vi "DPT Panel Volume Size.vi"(0 "Default Volume Value":dbl, 11 "Error In":errorcluster) -> (4 "Scale Temp Coeff Out":dbl, 6 "Drum Volume":dbl=6.0, 8 "Out Strings":string[][](array[string]), 10 "MA Filter Size":i32=5, 15 "Error Out":errorcluster)   [LabVIEW 2016]
uses:
  Utility/Custom Pallet Controls/Custom Pallet Forward.ctl
  Utility/Custom Pallet Controls/Custom Pallet DBL.ctl
panel:
  in  "Drum Thermal\nVolume (>0)":T1=13.0 format="%.2f"
  in  "Tab Control":enum32{"Page 1", "Page 2"}(tab)
  in  "MA Filter Size(>0)":string="40"
  in  "Scale Temp Coeff":string="0"
  in  "stop":T2
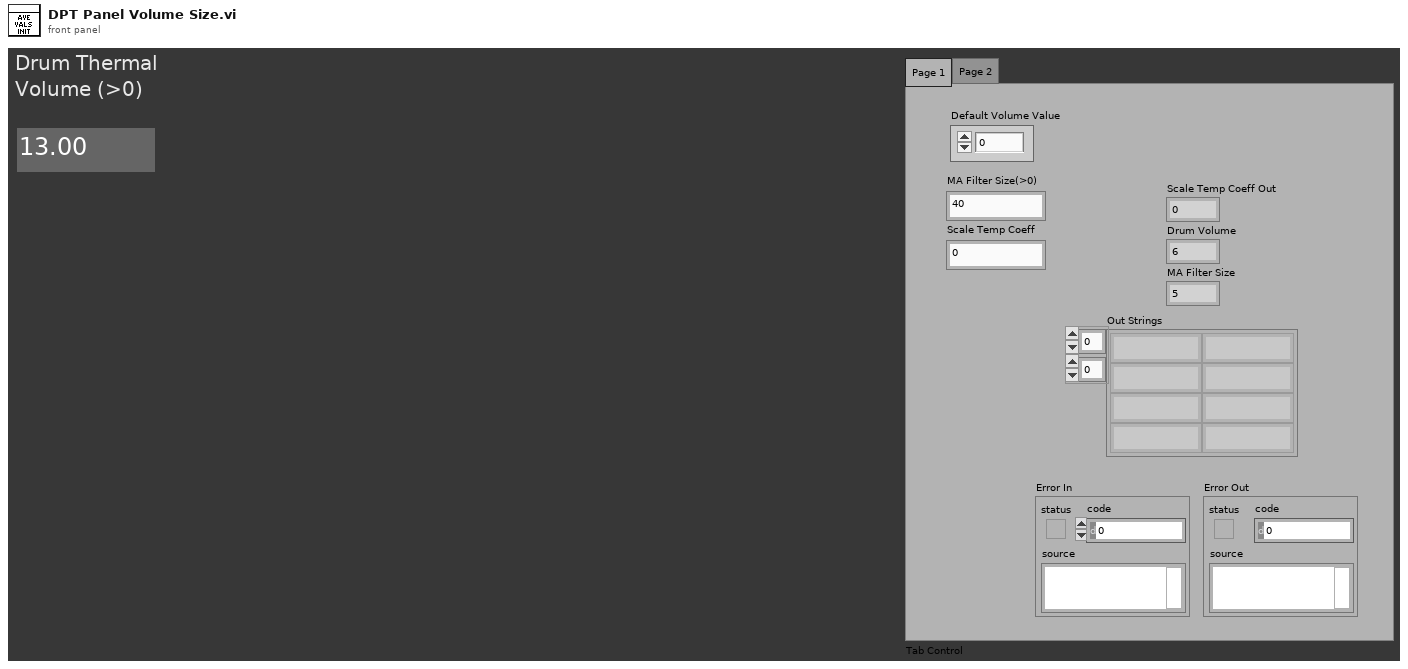
[diagram p1: front panel]
types:
  T1 = typedef "Custom Pallet DBL.ctl" = dbl
  T2 = typedef "Custom Pallet Forward.ctl" = bool
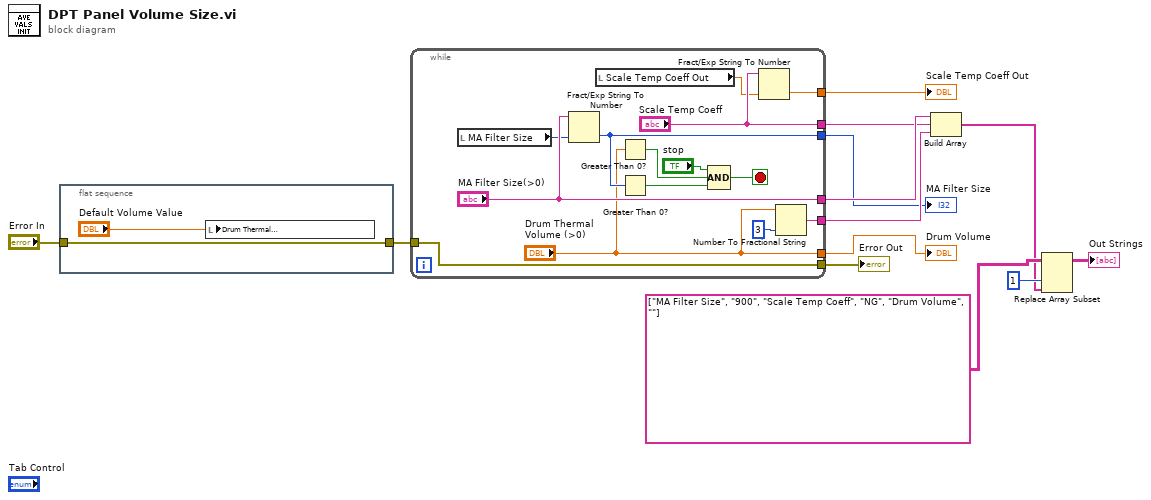
[diagram p0: block diagram]
diagram:
  n1 = flat-sequence {
    tunnel: "Error In" -> [w15]
    tunnel: [w15] -> w2
    frame #0 {
      n2 = local write "Drum Thermal\nVolume (>0)"("Default Volume Value") -> ()
    }
  }
  n3 = while {
    tunnel: ["MA Filter Size(>0)"] -> w11
    tunnel: ["Scale Temp Coeff"] -> w9
    tunnel: [w17] -> w8
    tunnel: [w22] -> w6
    tunnel: [w20] -> w5
    tunnel: ["Drum Thermal\nVolume (>0)"] -> w4
    tunnel: w2 -> [w16]
    tunnel: [w16] -> w1
    stop <- w24 stop-if-true
    n4 = local read "MA Filter Size"() -> (w23:i32)
    n5 = Fract/Exp String To Number(string="MA Filter Size(>0)", default (0 dbl)=w23) -> (number=w22:i32)  [unwired: 2 in, 1 out]
    n6 = local read "Scale Temp Coeff Out"() -> (w21:dbl)
    n7 = Greater Than 0?(x="Drum Thermal\nVolume (>0)") -> (x > 0?=w26:bool)
    n8 = Greater Than 0?(x=w22) -> (x > 0?=w25:bool)
    n9 = Compound Arithmetic op=AND("stop", w26, w25) -> (w24:T2)
    n10 = Fract/Exp String To Number(string="Scale Temp Coeff", default (0 dbl)=w21) -> (number=w20:dbl)  [unwired: 2 in, 1 out]
    n11 = Number To Fractional String(number="Drum Thermal\nVolume (>0)", precision (6)=i16 3) -> (F-format string=w17:string)  [unwired: 2 in]
  }
  "Error Out" <- w1
  "MA Filter Size" <- w6
  "Scale Temp Coeff Out" <- w5
  "Drum Volume" <- w4
  n12 = Build Array(w11, w9, w8) -> (w10:string[])
  n13 = Replace Array Subset(array=string[][] [["MA Filter Size", "900"], ["Scale Temp Coeff", "NG"], ["Drum Volume", ""]] ("appended array"), new element=w10, index (col)=1 ("disabled index (col)")) -> (→"Out Strings":string[][])  [unwired: 1 in]
